vi "Autonomous A3 Right-deliverswitch-move out of way.vi"   [LabVIEW 2017]
uses:
  Framework/Robot Global Data.vi
types:
  T1 = typedef "Command Status Info.ctl" = cluster{"Name":string, "Status":T2, "notifier out":T3}
  T2 = typedef "Completion Status.ctl" = enum16{"Successful", "Aborted", "Incomplete"}
  T3 = typedef "Completion Notifier.ctl" = refnum<notifier>
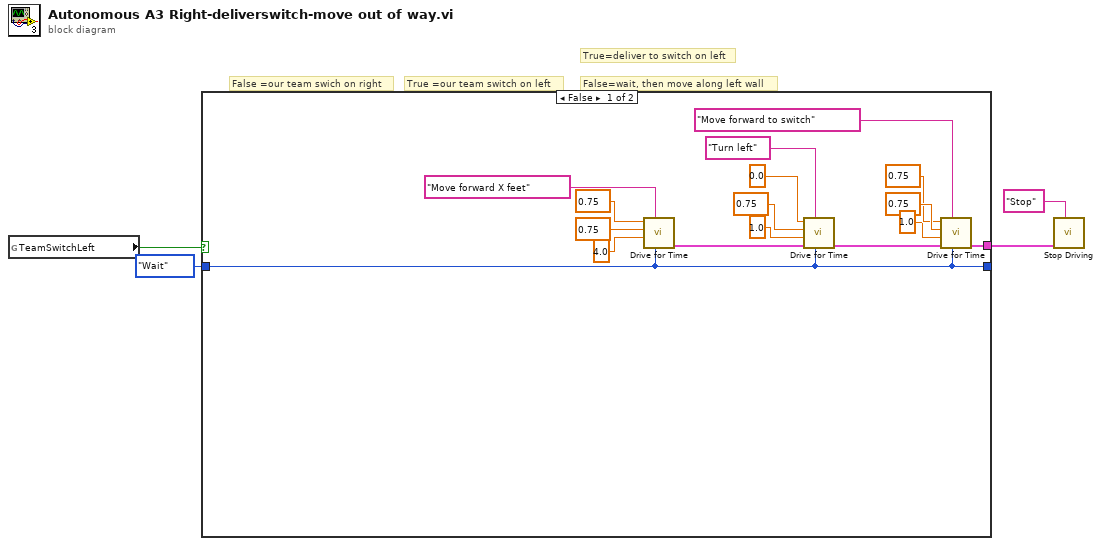
[diagram p0: block diagram]
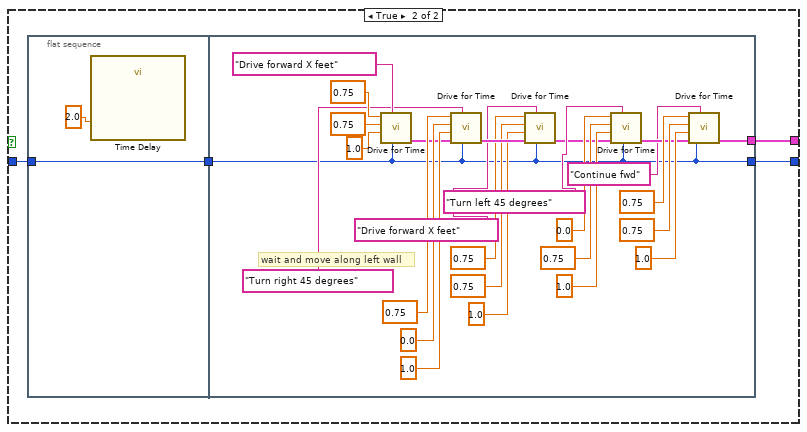
[diagram p2: hidden frame]
diagram:
  # "False=wait, then move along left wall"
  # "True=deliver to switch on left"
  # "False =our team swich on right"
  # "True =our team switch on left"
  n1 = global read "Robot Global Data.vi" "TeamSwitchLeft"() -> (w1:bool)
  n2 = case shown="False" w1 {
    tunnel: [w7 w24] -> w3
    tunnel: [w6 w21] -> _
    tunnel: enum16{"Start", "Wait"}."Wait" ("Synchronication") -> [w6 w23]
    frame False {
      n3 = call "Drive for Time.vi"("Synchronization"=w6, "Description"="Move forward X feet", "Seconds"=4.0, "Right Speed"=0.75, "Left Speed"=0.75) -> ("Command Info Out"=w5:T1)  [unwired: 5 in, 1 out]
      n4 = call "Drive for Time.vi"("Synchronization"=w6, "Description"="Turn left", "Command Info In"=w5, "Seconds"=1.0, "Right Speed"=0.75, "Left Speed"=0.0) -> ("Command Info Out"=w12:T1)  [unwired: 4 in, 1 out]
      n5 = call "Drive for Time.vi"("Synchronization"=w6, "Description"="Move forward to switch", "Command Info In"=w12, "Seconds"=1.0, "Right Speed"=0.75, "Left Speed"=0.75) -> ("Command Info Out"=w7:T1)  [unwired: 4 in, 1 out]
    }
    frame True {
      n6 = flat-sequence {
        tunnel: w23 -> [w25]
        tunnel: [w25] -> w22
        tunnel: [w29] -> w24
        tunnel: w22 -> [w27]
        tunnel: [w27] -> w21
        frame #0 {
          n7 = call "Time Delay"("Delay Time (s)"=2.0) -> ()  [unwired: 10 in, 1 out]
        }
        frame #1 {
          # "wait and move along left wall"
          n8 = call "Drive for Time.vi"("Synchronization"=w27, "Description"="Drive forward X feet", "Seconds"=1.0, "Right Speed"=0.75, "Left Speed"=0.75 ("Right Speed")) -> ("Command Info Out"=w45:T1)  [unwired: 5 in, 1 out]
          n9 = call "Drive for Time.vi"("Synchronization"=w27, "Description"="Turn right 45 degrees", "Command Info In"=w45, "Seconds"=1.0, "Right Speed"=0.0, "Left Speed"=0.75) -> ("Command Info Out"=w43:T1)  [unwired: 4 in, 1 out]
          n10 = call "Drive for Time.vi"("Synchronization"=w27, "Description"="Drive forward X feet", "Command Info In"=w43, "Seconds"=1.0, "Right Speed"=0.75, "Left Speed"=0.75 ("Right Speed")) -> ("Command Info Out"=w42:T1)  [unwired: 4 in, 1 out]
          n11 = call "Drive for Time.vi"("Synchronization"=w27, "Description"="Turn left 45 degrees", "Command Info In"=w42, "Seconds"=1.0, "Right Speed"=0.75, "Left Speed"=0.0) -> ("Command Info Out"=w30:T1)  [unwired: 4 in, 1 out]
          n12 = call "Drive for Time.vi"("Synchronization"=w27, "Description"="Continue fwd", "Command Info In"=w30, "Seconds"=1.0, "Right Speed"=0.75, "Left Speed"=0.75) -> ("Command Info Out"=w29:T1)  [unwired: 4 in, 1 out]
        }
      }
    }
  }
  n13 = call "Stop Driving.vi"("Description"="Stop", "Command Info In"=w3) -> ()  [unwired: 9 in, 1 out]
